vi "Remove_strings_fr_Array.vi"(1 "Input Strings":string[](array[string]), 2 "Strings to remove":string[](array[string])) -> (0 "Output Strings":string[](array[string]))   [LabVIEW 2010]
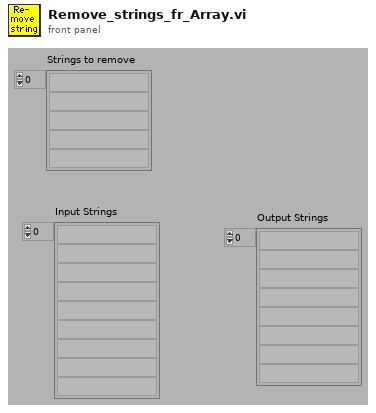
[diagram p1: front panel]
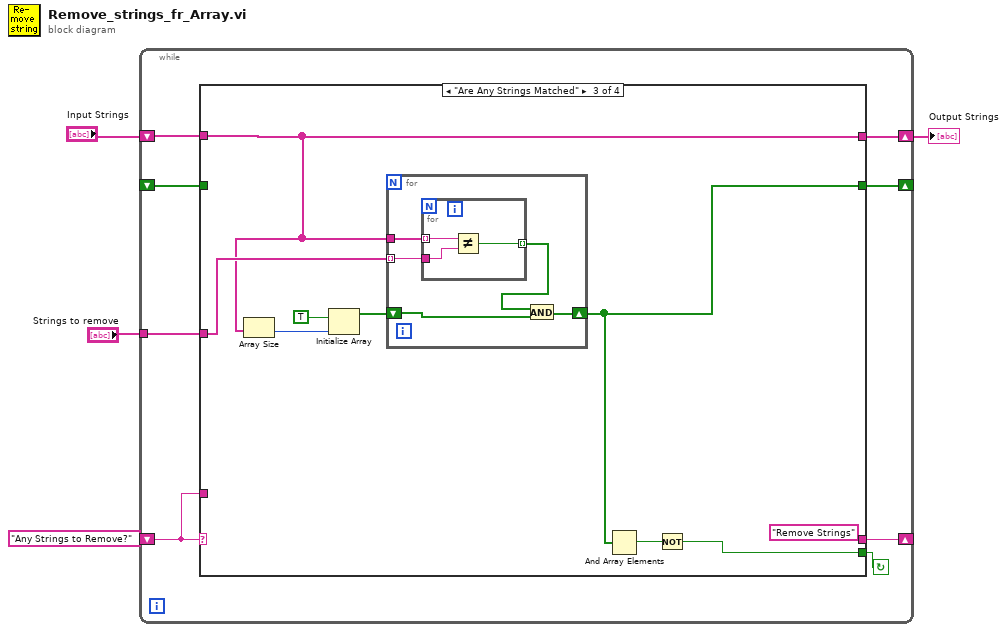
[diagram p0: block diagram]
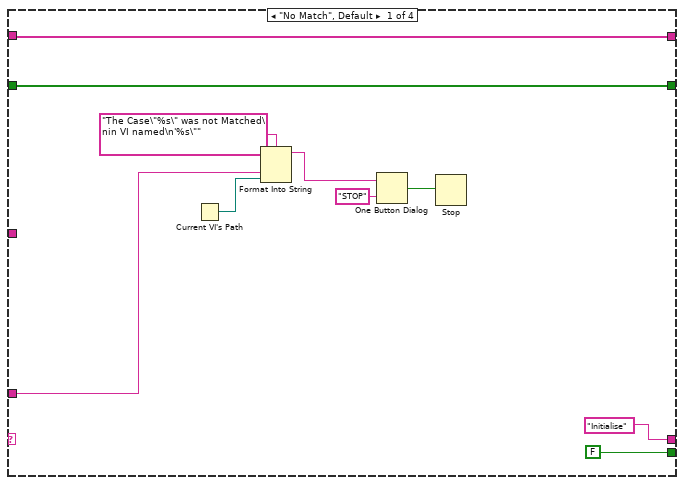
[diagram p2: hidden frame]
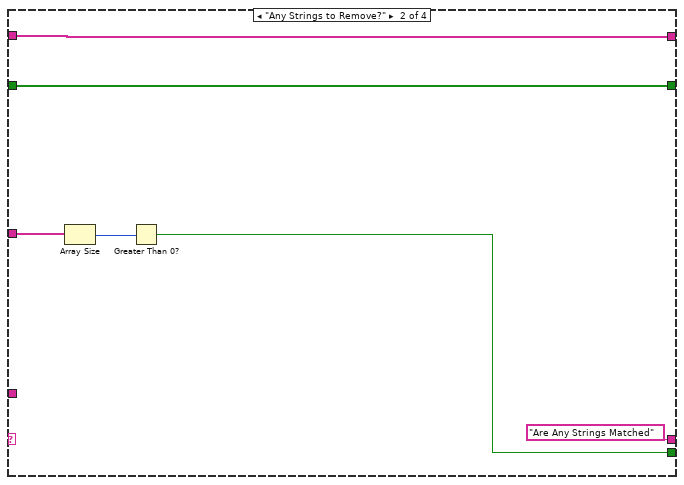
[diagram p3: hidden frame]
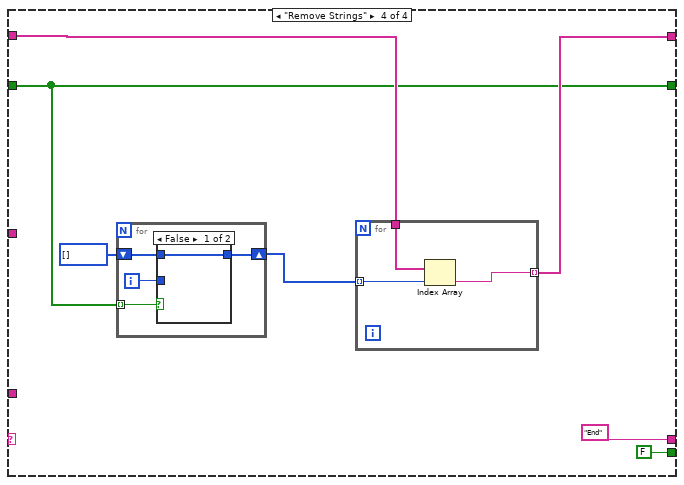
[diagram p4: hidden frame]
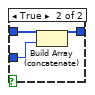
[diagram p5: hidden frame]
diagram:
  n1 = while {
    shift-left: _ -> [w5]
    shift-right: [w6] -> _
    tunnel: "Strings to remove" -> [w7]
    shift-left: "Input Strings" -> [w9]
    shift-right: [w8] -> w2
    shift-left: "Any Strings to Remove?" -> [w10]
    shift-right: [w11] -> _
    stop <- w12 continue-if-true
    n2 = case shown="\"Are Any Strings Matched\"" w10 {
      tunnel: [FALSE w25 w31 FALSE] -> w12
      tunnel: ["Initialise" "Are Any Strings Matched" "Remove Strings" "End"] -> w11
      tunnel: w10 -> [w17 _ _ _]
      tunnel: w9 -> [w14 w27 w30 w49]
      tunnel: [w14 w27 w30 w48] -> w8
      tunnel: w7 -> [_ w26 w36 _]
      tunnel: [w13 w24 w33 w47] -> w6
      tunnel: w5 -> [w13 w24 _ w47]
      frame "No Match", Default {
        n3 = Current VI's Path() -> (path=w16:path)
        n4 = Format Into String(format string="The Case\"%s\" was not Matched\nin VI named\n'%s\"" ("Format String"), w17, w16) -> (resulting string=w20:string)  [unwired: 2 in, 1 out]
        n5 = One Button Dialog(message=w20, button name ("OK")="STOP") -> (true=w18:bool)
        n6 = Stop(stop? (T)=w18) -> ()
      }
      frame "Any Strings to Remove?" {
        n7 = Array Size(array=w26) -> (size(s)=w23:i32)
        n8 = Greater Than 0?(x=w23) -> (x > 0?=w25:bool)
      }
      frame "Are Any Strings Matched" {
        n9 = Array Size(array=w30) -> (size(s)=w29:i32)
        n10 = Initialize Array(TRUE, w29) -> (w34:bool[])
        n11 = for {
          tunnel: w30 -> [w42]
          tunnel: w36 -> [w41] mode=indexing
          shift-right: [w38] -> w33
          shift-left: w34 -> [w40]
          n12 = for {
            tunnel: w42 -> [w45] mode=indexing
            tunnel: w41 -> [w44]
            tunnel: [w43] -> w39 mode=indexing
            n13 = Not Equal?(x=w45, y=w44) -> (x != y?=w43:bool)
          }
          n14 = And(x=w39, y=w40) -> (x .and. y?=w38:bool[])
        }
        n15 = And Array Elements(Boolean array=w33) -> (logical AND=w32:bool)
        n16 = Not(x=w32) -> (.not. x?=w31:bool)
      }
      frame "Remove Strings" {
        n17 = for {
          shift-right: [w57] -> w50
          shift-left: i32[] [] -> [w56]
          tunnel: w47 -> [w59] mode=indexing
          i -> [w58]
          n18 = case shown="False" w59 {
            tunnel: w58 -> [_ w62]
            tunnel: [w60 w61] -> w57
            tunnel: w56 -> [w60 w63]
            frame False {
            }
            frame True {
              n19 = Build Array (concatenate)(w63, w62) -> (w61:i32[])
            }
          }
        }
        n20 = for {
          tunnel: w50 -> [w55] mode=indexing
          tunnel: w49 -> [w54]
          tunnel: [w53] -> w48 mode=indexing
          n21 = Index Array(array=w54, index=w55) -> (element=w53:string)
        }
      }
    }
  }
  "Output Strings" <- w2
